vi "AddToTopicsGlobal.vi"(3 "ROS in":T1) -> (1 "ROS out":T1)   [LabVIEW 2012]
doc: "Adds a topic to the global topic list"
uses:
  _ROSDefinition.vi
  _ROSDirection.ctl
  _ROSControl.ctl
panel:
  out "new?":bool
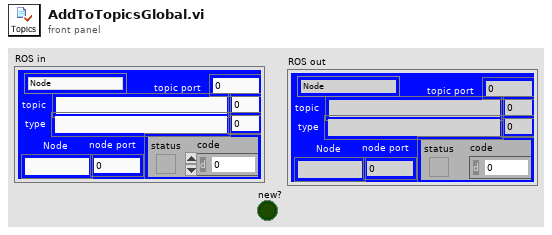
[diagram p1: front panel]
types:
  T1 = typedef "_ROSControl.ctl" = cluster{"topic port":u16, "Node":string, "topic":string, "type":string, "node port":u16, "error ":errorcluster, "Direction":T2, "Update (ms)":u16, "FIFO size":u16}
  T2 = typedef "_ROSDirection.ctl" = enum16{"Node", "Publisher", "Subscriber", "ServiceClient", "ServiceProvider"}
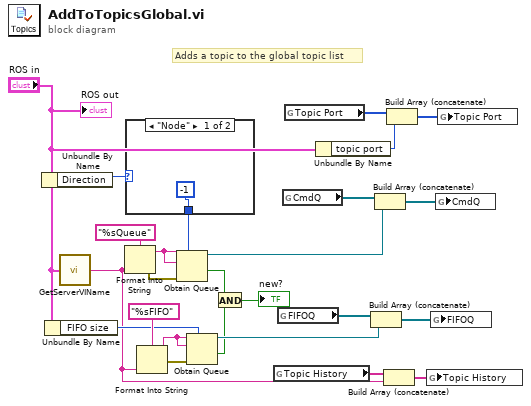
[diagram p0: block diagram]
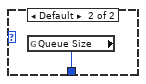
[diagram p2: hidden frame]
diagram:
  # "Adds a topic to the global topic list"
  n1 = Unbundle By Name("ROS in") -> ("Direction"=w1:T2)
  n2 = Unbundle By Name("ROS in") -> ("FIFO size"=w18:u16)
  n3 = call "GetServerVIName.vi"("ROS"="ROS in") -> ("vi name"=w17:string)
  n4 = Format Into String(format string="%sQueue" ("name (unnamed)"), w17) -> (resulting string=w23:string, error out=w24:errorcluster)  [unwired: 2 in]
  n5 = case shown="\"Node\"" w1 {
    tunnel: [-1 ("Queue Size") w27] -> w25
    frame "Node" {
    }
    frame Default {
      n6 = global read "_ROSDefinition.vi" "Queue Size"() -> (w27:i32)
    }
  }
  n7 = Format Into String(format string="%sFIFO" ("name (unnamed)"), w17) -> (resulting string=w19:string, error out=w20:errorcluster)  [unwired: 2 in]
  n8 = Obtain Queue(max queue size (-1, unlimited)=w25, name (unnamed)=w23, element data type=w23, error in (no error)=w24) -> (queue out=w16:refnum<queue>, created new?=w5:bool)  [unwired: 1 in, 1 out]
  n9 = Obtain Queue(max queue size (-1, unlimited)=w18, name (unnamed)=w19, element data type=w19, error in (no error)=w20) -> (queue out=w15:refnum<queue>, created new?=w4:bool)  [unwired: 1 in, 1 out]
  n10 = And(x=w5, y=w4) -> (x .and. y?=→"new?":bool)
  n11 = global read "_ROSDefinition.vi" "Topic History"() -> (w14:string[])
  n12 = global read "_ROSDefinition.vi" "FIFOQ"() -> (w6:refnum<queue>[])
  n13 = global read "_ROSDefinition.vi" "CmdQ"() -> (w9:refnum<queue>[])
  n14 = global read "_ROSDefinition.vi" "Topic Port"() -> (w11:u16[])
  n15 = Unbundle By Name("ROS in") -> ("topic port"=w10:u16)
  n16 = Build Array (concatenate)(w6, w15) -> (w7:refnum<queue>[])
  n17 = Build Array (concatenate)(w9, w16) -> (w8:refnum<queue>[])
  n18 = Build Array (concatenate)(w14, w17) -> (w13:string[])
  n19 = Build Array (concatenate)(w11, w10) -> (w12:u16[])
  n20 = global write "_ROSDefinition.vi" "Topic History"(w13) -> ()
  n21 = global write "_ROSDefinition.vi" "FIFOQ"(w7) -> ()
  n22 = global write "_ROSDefinition.vi" "CmdQ"(w8) -> ()
  n23 = global write "_ROSDefinition.vi" "Topic Port"(w12) -> ()
  "ROS out" <- "ROS in"
